vi "Reading shit.vi"() -> ()   [LabVIEW 2009]
panel:
  out "Read data":cluster{"Longitude":dbl, "Latitude":dbl}[](array[cluster])
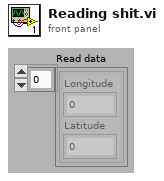
[diagram p1: front panel]
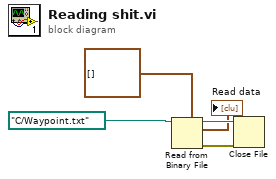
[diagram p0: block diagram]
diagram:
  n1 = Read from Binary File(5:cluster{"Longitude":dbl, "Latitude":dbl}[] [] ("Unsorted Waypoints"), 11:path "C:/Waypoint.txt" ("file path (use dialog)")) -> (0:w3:errorcluster, 2:→"Read data":cluster{"Longitude":dbl, "Latitude":dbl}[], 3:w2:refnum<file>)  [unwired: 4 in, 1 out]
  n2 = Close File(refnum=w2, error in=w3) -> ()  [unwired: 2 out]
